vi "Initialize Default Value.vi"(8 "error in (no error)":errorcluster, 11 "Numeric Data Type in":refnum<class "Numeric Data Type.lvclass">) -> (0 "error out":errorcluster, 3 "Numeric Data Type (dup)":refnum<class "Numeric Data Type.lvclass">)   [LabVIEW 2018, in "Numeric Data Type.lvclass"]
uses:
  Numeric Data Type.lvclass
  Numeric Data Type.lvclass/Numeric Data Type.ctl
  Reference Default Value (Complex).vi
  Reference Default Value.vi
  Reference Default Value (Date-Time).vi
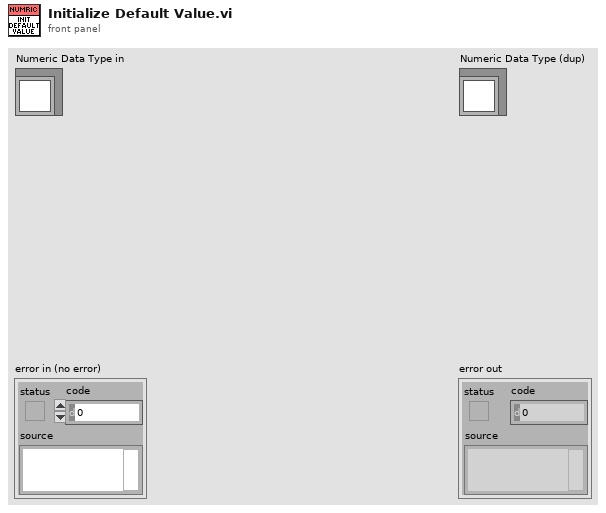
[diagram p1: front panel]
types:
  T1 = typedef "Numeric Data Type.lvclass/Representation Enum.ctl" = enum16{"Extended (EXT)", "Double (DBL)", "Single (SGL)", "Fixed-Point (FXP)", "Quad Integer (I64)", "Long Integer (I32)", "Word Integer (I16)", "Byte Integer (I8)", "Unsigned Quad (U64)", "Unsigned Long (U32)", "Unsigned Word (U16)", "Unsigned Byte (U8)", "Complex Extended (CXT)", "Complex Double (CDB)", "Complex Single (CSG)"}
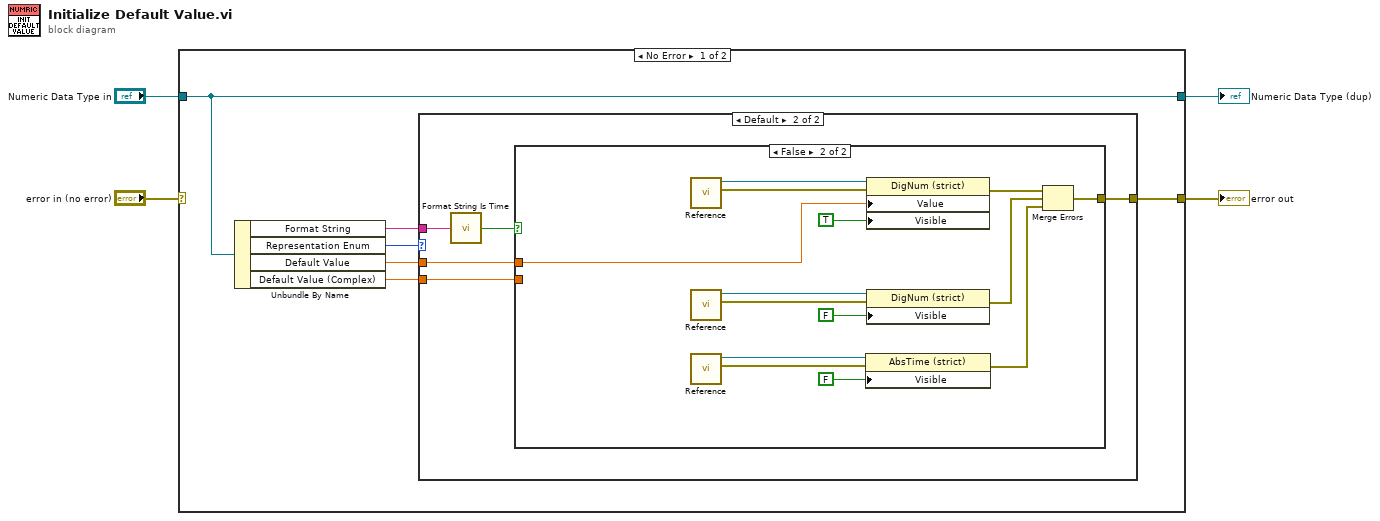
[diagram p0: block diagram]
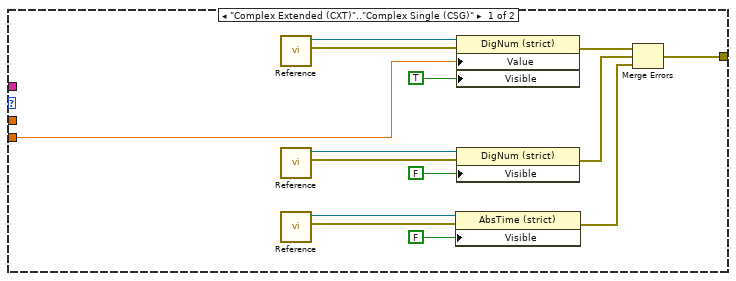
[diagram p2: hidden frame]
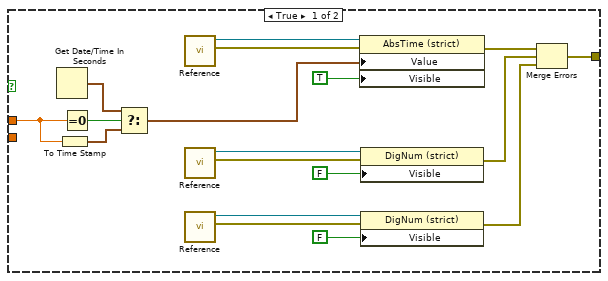
[diagram p3: hidden frame]
diagram:
  n1 = case shown="No Error" "error in (no error)" {
    selector: "error in (no error)" -> [_ w63]
    tunnel: [w5 w63] -> w3
    tunnel: [w10 w62] -> w1
    tunnel: "Numeric Data Type in" -> [w10 w62]
    frame No Error {
      n2 = Unbundle By Name(w10) -> ("Format String"=w6:string, "Representation Enum"=w9:T1, "Default Value"=w8:dbl, "Default Value (Complex)"=w7:cdb)
      n3 = case shown="Default" w9 {
        tunnel: w8 -> [_ w26]
        tunnel: w7 -> [w23 w29]
        tunnel: w6 -> [_ w28]
        tunnel: [w11 w25] -> w5
        frame "Complex Extended (CXT)".."Complex Single (CSG)" {
          n4 = call-poly "Reference.vi"() -> ("error out"=w16:errorcluster, "Default Value"=w24:refnum<vi>)  [unwired: 10 in]
          n5 = call-poly "Reference.vi"() -> ("error out"=w17:errorcluster, "Default Value"=w22:refnum<vi>)  [unwired: 10 in]
          n6 = call-poly "Reference.vi"() -> ("error out"=w15:errorcluster, "Default Value"=w18:refnum<vi>)  [unwired: 10 in]
          n7 = property class="AbsTime (strict)"(reference=w18, error in=w15, "Visible"=FALSE) -> (error out=w12:errorcluster)  [unwired: 1 out]
          n8 = property class="DigNum (strict)"(reference=w24, error in=w16, "Value"=w23, "Visible"=TRUE) -> (error out=w14:errorcluster)  [unwired: 1 out]
          n9 = property class="DigNum (strict)"(reference=w22, error in=w17, "Visible"=FALSE) -> (error out=w13:errorcluster)  [unwired: 1 out]
          n10 = Merge Errors(w14, w13, w12) -> (w11:errorcluster)
        }
        frame Default {
          n11 = call "Format String Is Time.vi"("Format String"=w28) -> ("Time?"=w27:bool)
          n12 = case shown="False" w27 {
            tunnel: w29 -> [_ _]
            tunnel: w26 -> [w33 w52]
            tunnel: [w35 w48] -> w25
            frame True {
              n13 = Get Date/Time In Seconds() -> (seconds since 1Jan1904=w31:timestamp)
              n14 = To Time Stamp(1:w33) -> (0:w32:timestamp)
              n15 = Equal To 0?(x=w33) -> (x = 0?=w34:bool)
              n16 = Select(t=w31, s=w34, f=w32) -> (s? t:f=w30:timestamp)
              n17 = call-poly "Reference.vi"() -> ("error out"=w40:errorcluster, "Default Value"=w47:refnum<vi>)  [unwired: 10 in]
              n18 = call-poly "Reference.vi"() -> ("error out"=w41:errorcluster, "Default Value"=w46:refnum<vi>)  [unwired: 10 in]
              n19 = call-poly "Reference.vi"() -> ("error out"=w39:errorcluster, "Default Value"=w42:refnum<vi>)  [unwired: 10 in]
              n20 = property class="AbsTime (strict)"(reference=w47, error in=w40, "Value"=w30, "Visible"=TRUE) -> (error out=w38:errorcluster)  [unwired: 1 out]
              n21 = property class="DigNum (strict)"(reference=w46, error in=w41, "Visible"=FALSE) -> (error out=w37:errorcluster)  [unwired: 1 out]
              n22 = property class="DigNum (strict)"(reference=w42, error in=w39, "Visible"=FALSE) -> (error out=w36:errorcluster)  [unwired: 1 out]
              n23 = Merge Errors(w38, w37, w36) -> (w35:errorcluster)
            }
            frame False {
              n24 = call-poly "Reference.vi"() -> ("error out"=w54:errorcluster, "Default Value"=w61:refnum<vi>)  [unwired: 10 in]
              n25 = call-poly "Reference.vi"() -> ("error out"=w55:errorcluster, "Default Value"=w60:refnum<vi>)  [unwired: 10 in]
              n26 = call-poly "Reference.vi"() -> ("error out"=w53:errorcluster, "Default Value"=w56:refnum<vi>)  [unwired: 10 in]
              n27 = property class="AbsTime (strict)"(reference=w56, error in=w53, "Visible"=FALSE) -> (error out=w49:errorcluster)  [unwired: 1 out]
              n28 = property class="DigNum (strict)"(reference=w61, error in=w54, "Value"=w52, "Visible"=TRUE) -> (error out=w51:errorcluster)  [unwired: 1 out]
              n29 = property class="DigNum (strict)"(reference=w60, error in=w55, "Visible"=FALSE) -> (error out=w50:errorcluster)  [unwired: 1 out]
              n30 = Merge Errors(w51, w50, w49) -> (w48:errorcluster)
            }
          }
        }
      }
    }
    frame Error {
    }
  }
  "error out" <- w3
  "Numeric Data Type (dup)" <- w1
